vi "CRake Learn Template.vi"(8 "error in":errorcluster, 9 "Image in":T1, 10 "Template details":T2={"Process parameters"={"ROI parameters"={"Step Size"=20, "r offset"=10, "Edge Options"={"Edge Polarity"=0, "Kernel Size"=7, "Width"=5, "Minimum Edge Strength"=100.0, "Interpolation Type"=enum."Bilinear Fixed", "Data Processing Method"=enum."Average"}, "Annulus\ndetails"={"Center X"=0, "Center Y"=0, "Inner Radius"=0, "Outer Radius"=3900, "Start Angle"=0.0, "End Angle"=0.0}}, "Dust removal details"={"Remove dust"=TRUE, "Dust removal data"={"Dilate data"={"Operation"=enum."Erode", "Structuring Element"=[[1, 1, 1], [1, 1, 1], [1, 1, 1]], "Number of iterations (1)"=3, "Square/Hexa (Square)"=TRUE}, "Threshold data"={"Method (clustering)"=0, "Look For (Bright Objects)"=1, "Range"={"Lower value"=128.0, "Upper value"=255.0}, "Replace Value"=255.0}}}}, "LearningData"={"Angle info"={"Rising edge angles"=[{"Edge angles"=[]}, {"Edge angles"=[]}, {"Edge angles"=[]}, {"Edge angles"=[]}, {"Edge angles"=[]}, {"Edge angles"=[]}, {"Edge angles"=[]}, {"Edge angles"=[]}, {"Edge angles"=[]}, {"Edge angles"=[]}, {"Edge angles"=[]}, {"Edge angles"=[]}, {"Edge angles"=[]}, {"Edge angles"=[]}, {"Edge angles"=[324.4002990722656, 279.37237548828125, 234.31814575195312, 189.45828247070312, 144.43719482421875, 99.26164245605469, 54.478885650634766, 9.288665771484375]}, {"Edge angles"=[326.8953857421875, 282.0519714355469, 237.04156494140625, 192.0699920654297, 147.00604248046875, 102.04810333251953, 57.04718017578125, 12.020856857299805]}, {"Edge angles"=[327.23541259765625, 282.35137939453125, 237.37074279785156, 192.36749267578125, 147.3665313720703, 102.35699462890625, 57.358543395996094, 12.353824615478516]}, {"Edge angles"=[357.3017883300781, 326.07904052734375, 281.0994567871094, 236.0724639892578, 235.6566925048828, 191.1215057373047, 146.08834838867188, 101.15013122558594, 56.03056716918945, 11.077372550964355]}, {"Edge angles"=[322.224609375, 277.2630615234375, 232.26690673828125, 96.92642974853516, 52.116703033447266, 7.029767990112305]}, {"Edge angles"=[]}, {"Edge angles"=[]}, {"Edge angles"=[]}, {"Edge angles"=[]}, {"Edge angles"=[]}, {"Edge angles"=[]}, {"Edge angles"=[]}, {"Edge angles"=[356.58099365234375, 350.285400390625, 343.9516296386719, 337.64874267578125, 331.33636474609375, 325.0185241699219, 318.6827697753906, 312.3748779296875, 306.0724792480469, 299.736083984375, 293.4723815917969, 287.15020751953125, 280.8420715332031, 274.51861572265625, 268.1320495605469, 261.8740539550781, 255.5738983154297, 249.276123046875, 242.95098876953125, 236.62612915039062, 230.31637573242188, 224.009521484375, 217.69149780273438, 211.35440063476562, 205.0513916015625, 198.69039916992188, 192.43421936035156, 186.09483337402344, 179.81744384765625, 173.4593505859375, 167.0970001220703, 160.7847900390625, 154.46017456054688, 148.13107299804688, 141.8062286376953, 135.53399658203125, 129.20545959472656, 122.88826751708984, 116.5517349243164, 110.27731323242188, 103.95439910888672, 97.63215637207031, 91.3005142211914, 85.0173568725586, 78.71366119384766, 72.41765594482422, 65.96402740478516, 59.750633239746094, 53.4320068359375, 47.08340835571289, 40.791725158691406, 34.49047088623047, 28.16463851928711, 21.869430541992188, 15.541481018066406, 9.238995552062988, 2.9198527336120605]}, {"Edge angles"=[357.50360107421875, 351.15313720703125, 344.8380432128906, 338.5302429199219, 332.2137756347656, 325.804443359375, 319.57830810546875, 313.2322998046875, 306.92938232421875, 300.63079833984375, 294.3407287597656, 288.0224304199219, 281.7042236328125, 275.3729248046875, 269.0707702636719, 262.775390625, 256.4610900878906, 250.14210510253906, 243.842529296875, 237.52635192871094, 231.20989990234375, 224.88641357421875, 218.57626342773438, 212.2597198486328, 205.92007446289062, 199.60572814941406, 193.28834533691406, 186.9896240234375, 180.66493225097656, 174.3603057861328, 168.0143280029297, 161.70201110839844, 155.35635375976562, 149.0479278564453, 142.74942016601562, 136.41973876953125, 130.07635498046875, 123.77355194091797, 117.44210815429688, 111.15596771240234, 104.81024932861328, 98.50434875488281, 92.1738510131836, 85.8763427734375, 79.58023071289062, 73.2815170288086, 66.96917724609375, 60.62763595581055, 54.32320785522461, 48.03331756591797, 41.69807434082031, 35.39656066894531, 29.04926872253418, 22.751008987426758, 16.438982009887695, 10.120953559875488, 3.7855653762817383]}], "Falling edge angles"=[{"Edge angles"=[]}, {"Edge angles"=[]}, {"Edge angles"=[]}, {"Edge angles"=[]}, {"Edge angles"=[]}, {"Edge angles"=[]}, {"Edge angles"=[]}, {"Edge angles"=[]}, {"Edge angles"=[]}, {"Edge angles"=[]}, {"Edge angles"=[]}, {"Edge angles"=[]}, {"Edge angles"=[]}, {"Edge angles"=[]}, {"Edge angles"=[358.7027587890625, 313.5650939941406, 268.6748962402344, 223.70919799804688, 178.54701232910156, 133.67933654785156, 88.60447692871094, 43.56612777709961]}, {"Edge angles"=[355.9402770996094, 310.9671325683594, 266.03912353515625, 221.030029296875, 175.98460388183594, 130.972412109375, 86.0030517578125, 40.94852828979492]}, {"Edge angles"=[355.5914611816406, 310.6212463378906, 265.676513671875, 220.6667022705078, 175.67599487304688, 130.68984985351562, 85.72019958496094, 40.68776321411133]}, {"Edge angles"=[357.8193054199219, 357.139404296875, 311.851318359375, 266.9569091796875, 235.827880859375, 221.9400177001953, 176.938232421875, 131.88555908203125, 86.9477310180664, 41.9368782043457]}, {"Edge angles"=[315.7031555175781, 225.93267822265625, 180.75328063964844, 135.82232666015625, 46.085636138916016, 0.9171632528305054]}, {"Edge angles"=[]}, {"Edge angles"=[]}, {"Edge angles"=[]}, {"Edge angles"=[]}, {"Edge angles"=[]}, {"Edge angles"=[]}, {"Edge angles"=[]}, {"Edge angles"=[354.0222473144531, 347.68878173828125, 341.4031677246094, 335.0976257324219, 328.770263671875, 322.4639892578125, 316.15887451171875, 309.8772277832031, 303.5346984863281, 297.2074890136719, 290.9279479980469, 284.62744140625, 278.2616882324219, 271.9461669921875, 265.6507568359375, 259.335205078125, 253.01336669921875, 246.688720703125, 240.3791961669922, 234.10598754882812, 227.7845001220703, 221.4361114501953, 215.10934448242188, 208.79022216796875, 202.47589111328125, 196.1585235595703, 189.9136505126953, 183.51986694335938, 177.2025604248047, 170.8728485107422, 164.5511932373047, 158.22274780273438, 151.91403198242188, 145.59686279296875, 139.29791259765625, 132.97251892089844, 126.62997436523438, 120.33435821533203, 114.02253723144531, 107.7345199584961, 101.3875503540039, 95.11666107177734, 88.78436279296875, 82.45806884765625, 76.13545227050781, 69.85616302490234, 63.47029113769531, 57.14175796508789, 50.845458984375, 44.541873931884766, 38.223140716552734, 31.949254989624023, 25.62628746032715, 19.294870376586914, 12.989399909973145, 6.6459808349609375, 0.32935503125190735]}, {"Edge angles"=[359.45294189453125, 353.155517578125, 346.8225402832031, 340.52154541015625, 334.2013854980469, 327.8995361328125, 321.5911865234375, 315.29925537109375, 308.96868896484375, 302.6675720214844, 296.33758544921875, 290.021728515625, 283.70550537109375, 277.3900451660156, 271.0820007324219, 264.7945556640625, 258.4638366699219, 252.13612365722656, 245.82635498046875, 239.5060272216797, 233.20834350585938, 226.8910675048828, 220.53424072265625, 214.2158203125, 207.89846801757812, 201.5936279296875, 195.26161193847656, 188.94100952148438, 182.6217803955078, 176.31558227539062, 169.99583435058594, 163.67674255371094, 157.3478240966797, 151.02032470703125, 144.70858764648438, 138.41078186035156, 132.12911987304688, 125.7828140258789, 119.45489501953125, 113.16563415527344, 106.87589263916016, 100.5637435913086, 94.23698425292969, 87.91885375976562, 81.59281921386719, 75.27478790283203, 68.95628356933594, 62.62395477294922, 56.29034423828125, 49.94796371459961, 43.6364631652832, 37.34098815917969, 31.032493591308594, 24.706125259399414, 18.384830474853516, 12.063972473144531, 5.750241279602051]}]}, "Center"={"X"=5341.767, "Y"=4601.92}}, "Fine search details"={"FS angle range\n(in degrees)"=5.0, "FS angle step size\n(in degrees)"=0.001}, "Auto ROI detect"=TRUE} {"Process parameters"."ROI parameters"."Edge Options"."Edge Polarity" items=["All Edges", "Rising Edges", "Falling Edges"]; "Process parameters"."ROI parameters"."Edge Options"."Minimum Edge Strength" format="%.2f"; "Process parameters"."ROI parameters"."Edge Options"."Width" step=2; "Process parameters"."ROI parameters"."Edge Options"."Kernel Size" step=2; "Process parameters"."ROI parameters"."Annulus\ndetails"."End Angle" min=-90.0 max=90.0 step=1.0 format="%.2f"; "Process parameters"."ROI parameters"."Annulus\ndetails"."Start Angle" min=-90.0 max=90.0 step=1.0 format="%.2f"; "Process parameters"."ROI parameters"."Annulus\ndetails"."Center X" scale=0.0..1024.0; "Process parameters"."Dust removal details"."Dust removal data"."Threshold data"."Method (clustering)" items=["clustering", "entropy", "metric", "moments", "inter-class variance"]; "Process parameters"."Dust removal details"."Dust removal data"."Threshold data"."Look For (Bright Objects)" items=["Bright Objects", "Dark Objects"]}, 11 "Write parameters":T7={"Part name"="", "TemplateImage filepath"=path "E:/Algorithm/Geometric template matching/Images/Test images/Partially symmetric part/Part 1/Coarse angle/41.000000.png", "Template config filepath"=path "", "Testing?"=FALSE}) -> (0 "error out":errorcluster, 2 "Image indicator":T1(plugin-control), 3 "Template details out":T2={"Process parameters"={"ROI parameters"={"Step Size"=75, "r offset"=0, "Edge Options"={"Edge Polarity"=0, "Kernel Size"=0, "Width"=10, "Minimum Edge Strength"=2800.0, "Interpolation Type"=enum."Zero Order", "Data Processing Method"=enum."Average"}, "Annulus\ndetails"={"Center X"=0, "Center Y"=0, "Inner Radius"=0, "Outer Radius"=0, "Start Angle"=0.0, "End Angle"=0.0}}, "Dust removal details"={"Remove dust"=FALSE, "Dust removal data"={"Dilate data"={"Operation"=enum."Erode", "Structuring Element"=[[1, 1, 1], [1, 1, 1], [1, 1, 1]], "Number of iterations (1)"=5, "Square/Hexa (Square)"=TRUE}, "Threshold data"={"Method (clustering)"=0, "Look For (Bright Objects)"=1, "Range"={"Lower value"=128.0, "Upper value"=255.0}, "Replace Value"=255.0}}}}, "LearningData"={"Angle info"={"Rising edge angles"=[{"Edge angles"=[]}, {"Edge angles"=[]}, {"Edge angles"=[]}, {"Edge angles"=[]}, {"Edge angles"=[]}, {"Edge angles"=[]}, {"Edge angles"=[]}, {"Edge angles"=[]}, {"Edge angles"=[]}, {"Edge angles"=[]}, {"Edge angles"=[]}, {"Edge angles"=[]}, {"Edge angles"=[]}, {"Edge angles"=[]}, {"Edge angles"=[324.4002990722656, 279.37237548828125, 234.31814575195312, 189.45828247070312, 144.43719482421875, 99.26164245605469, 54.478885650634766, 9.288665771484375]}, {"Edge angles"=[326.8953857421875, 282.0519714355469, 237.04156494140625, 192.0699920654297, 147.00604248046875, 102.04810333251953, 57.04718017578125, 12.020856857299805]}, {"Edge angles"=[327.23541259765625, 282.35137939453125, 237.37074279785156, 192.36749267578125, 147.3665313720703, 102.35699462890625, 57.358543395996094, 12.353824615478516]}, {"Edge angles"=[357.3017883300781, 326.07904052734375, 281.0994567871094, 236.0724639892578, 235.6566925048828, 191.1215057373047, 146.08834838867188, 101.15013122558594, 56.03056716918945, 11.077372550964355]}, {"Edge angles"=[322.224609375, 277.2630615234375, 232.26690673828125, 96.92642974853516, 52.116703033447266, 7.029767990112305]}, {"Edge angles"=[]}, {"Edge angles"=[]}, {"Edge angles"=[]}, {"Edge angles"=[]}, {"Edge angles"=[]}, {"Edge angles"=[]}, {"Edge angles"=[]}, {"Edge angles"=[356.58099365234375, 350.285400390625, 343.9516296386719, 337.64874267578125, 331.33636474609375, 325.0185241699219, 318.6827697753906, 312.3748779296875, 306.0724792480469, 299.736083984375, 293.4723815917969, 287.15020751953125, 280.8420715332031, 274.51861572265625, 268.1320495605469, 261.8740539550781, 255.5738983154297, 249.276123046875, 242.95098876953125, 236.62612915039062, 230.31637573242188, 224.009521484375, 217.69149780273438, 211.35440063476562, 205.0513916015625, 198.69039916992188, 192.43421936035156, 186.09483337402344, 179.81744384765625, 173.4593505859375, 167.0970001220703, 160.7847900390625, 154.46017456054688, 148.13107299804688, 141.8062286376953, 135.53399658203125, 129.20545959472656, 122.88826751708984, 116.5517349243164, 110.27731323242188, 103.95439910888672, 97.63215637207031, 91.3005142211914, 85.0173568725586, 78.71366119384766, 72.41765594482422, 65.96402740478516, 59.750633239746094, 53.4320068359375, 47.08340835571289, 40.791725158691406, 34.49047088623047, 28.16463851928711, 21.869430541992188, 15.541481018066406, 9.238995552062988, 2.9198527336120605]}, {"Edge angles"=[357.50360107421875, 351.15313720703125, 344.8380432128906, 338.5302429199219, 332.2137756347656, 325.804443359375, 319.57830810546875, 313.2322998046875, 306.92938232421875, 300.63079833984375, 294.3407287597656, 288.0224304199219, 281.7042236328125, 275.3729248046875, 269.0707702636719, 262.775390625, 256.4610900878906, 250.14210510253906, 243.842529296875, 237.52635192871094, 231.20989990234375, 224.88641357421875, 218.57626342773438, 212.2597198486328, 205.92007446289062, 199.60572814941406, 193.28834533691406, 186.9896240234375, 180.66493225097656, 174.3603057861328, 168.0143280029297, 161.70201110839844, 155.35635375976562, 149.0479278564453, 142.74942016601562, 136.41973876953125, 130.07635498046875, 123.77355194091797, 117.44210815429688, 111.15596771240234, 104.81024932861328, 98.50434875488281, 92.1738510131836, 85.8763427734375, 79.58023071289062, 73.2815170288086, 66.96917724609375, 60.62763595581055, 54.32320785522461, 48.03331756591797, 41.69807434082031, 35.39656066894531, 29.04926872253418, 22.751008987426758, 16.438982009887695, 10.120953559875488, 3.7855653762817383]}], "Falling edge angles"=[{"Edge angles"=[]}, {"Edge angles"=[]}, {"Edge angles"=[]}, {"Edge angles"=[]}, {"Edge angles"=[]}, {"Edge angles"=[]}, {"Edge angles"=[]}, {"Edge angles"=[]}, {"Edge angles"=[]}, {"Edge angles"=[]}, {"Edge angles"=[]}, {"Edge angles"=[]}, {"Edge angles"=[]}, {"Edge angles"=[]}, {"Edge angles"=[358.7027587890625, 313.5650939941406, 268.6748962402344, 223.70919799804688, 178.54701232910156, 133.67933654785156, 88.60447692871094, 43.56612777709961]}, {"Edge angles"=[355.9402770996094, 310.9671325683594, 266.03912353515625, 221.030029296875, 175.98460388183594, 130.972412109375, 86.0030517578125, 40.94852828979492]}, {"Edge angles"=[355.5914611816406, 310.6212463378906, 265.676513671875, 220.6667022705078, 175.67599487304688, 130.68984985351562, 85.72019958496094, 40.68776321411133]}, {"Edge angles"=[357.8193054199219, 357.139404296875, 311.851318359375, 266.9569091796875, 235.827880859375, 221.9400177001953, 176.938232421875, 131.88555908203125, 86.9477310180664, 41.9368782043457]}, {"Edge angles"=[315.7031555175781, 225.93267822265625, 180.75328063964844, 135.82232666015625, 46.085636138916016, 0.9171632528305054]}, {"Edge angles"=[]}, {"Edge angles"=[]}, {"Edge angles"=[]}, {"Edge angles"=[]}, {"Edge angles"=[]}, {"Edge angles"=[]}, {"Edge angles"=[]}, {"Edge angles"=[354.0222473144531, 347.68878173828125, 341.4031677246094, 335.0976257324219, 328.770263671875, 322.4639892578125, 316.15887451171875, 309.8772277832031, 303.5346984863281, 297.2074890136719, 290.9279479980469, 284.62744140625, 278.2616882324219, 271.9461669921875, 265.6507568359375, 259.335205078125, 253.01336669921875, 246.688720703125, 240.3791961669922, 234.10598754882812, 227.7845001220703, 221.4361114501953, 215.10934448242188, 208.79022216796875, 202.47589111328125, 196.1585235595703, 189.9136505126953, 183.51986694335938, 177.2025604248047, 170.8728485107422, 164.5511932373047, 158.22274780273438, 151.91403198242188, 145.59686279296875, 139.29791259765625, 132.97251892089844, 126.62997436523438, 120.33435821533203, 114.02253723144531, 107.7345199584961, 101.3875503540039, 95.11666107177734, 88.78436279296875, 82.45806884765625, 76.13545227050781, 69.85616302490234, 63.47029113769531, 57.14175796508789, 50.845458984375, 44.541873931884766, 38.223140716552734, 31.949254989624023, 25.62628746032715, 19.294870376586914, 12.989399909973145, 6.6459808349609375, 0.32935503125190735]}, {"Edge angles"=[359.45294189453125, 353.155517578125, 346.8225402832031, 340.52154541015625, 334.2013854980469, 327.8995361328125, 321.5911865234375, 315.29925537109375, 308.96868896484375, 302.6675720214844, 296.33758544921875, 290.021728515625, 283.70550537109375, 277.3900451660156, 271.0820007324219, 264.7945556640625, 258.4638366699219, 252.13612365722656, 245.82635498046875, 239.5060272216797, 233.20834350585938, 226.8910675048828, 220.53424072265625, 214.2158203125, 207.89846801757812, 201.5936279296875, 195.26161193847656, 188.94100952148438, 182.6217803955078, 176.31558227539062, 169.99583435058594, 163.67674255371094, 157.3478240966797, 151.02032470703125, 144.70858764648438, 138.41078186035156, 132.12911987304688, 125.7828140258789, 119.45489501953125, 113.16563415527344, 106.87589263916016, 100.5637435913086, 94.23698425292969, 87.91885375976562, 81.59281921386719, 75.27478790283203, 68.95628356933594, 62.62395477294922, 56.29034423828125, 49.94796371459961, 43.6364631652832, 37.34098815917969, 31.032493591308594, 24.706125259399414, 18.384830474853516, 12.063972473144531, 5.750241279602051]}]}, "Center"={"X"=5341.767, "Y"=4601.92}}, "Fine search details"={"FS angle range\n(in degrees)"=5.0, "FS angle step size\n(in degrees)"=0.01}, "Auto ROI detect"=TRUE} {"Process parameters"."ROI parameters"."Edge Options"."Edge Polarity" items=["All Edges", "Rising Edges", "Falling Edges"]; "Process parameters"."ROI parameters"."Edge Options"."Minimum Edge Strength" format="%.2f"; "Process parameters"."ROI parameters"."Edge Options"."Width" step=2; "Process parameters"."ROI parameters"."Edge Options"."Kernel Size" step=2; "Process parameters"."ROI parameters"."Annulus\ndetails"."End Angle" min=-90.0 max=90.0 step=1.0 format="%.2f"; "Process parameters"."ROI parameters"."Annulus\ndetails"."Start Angle" min=-90.0 max=90.0 step=1.0 format="%.2f"; "Process parameters"."ROI parameters"."Annulus\ndetails"."Center X" scale=0.0..1024.0; "Process parameters"."Dust removal details"."Dust removal data"."Threshold data"."Method (clustering)" items=["clustering", "entropy", "metric", "moments", "inter-class variance"]; "Process parameters"."Dust removal details"."Dust removal data"."Threshold data"."Look For (Bright Objects)" items=["Bright Objects", "Dark Objects"]})   [LabVIEW 2015]
uses:
  CRake Pattern Matching/Controls/JSON parameters.ctl
  CRake Pattern Matching/Controls/ROI parameters.ctl
  <vilib>/vision/Measure.llb/Edge Options.ctl
  <vilib>/vision/Measure.llb/Edge Polarity.ctl
  <vilib>/vision/Image Controls.llb/IMAQ Image.ctl
panel:
  out "Image indicator 2":T1(plugin-control)
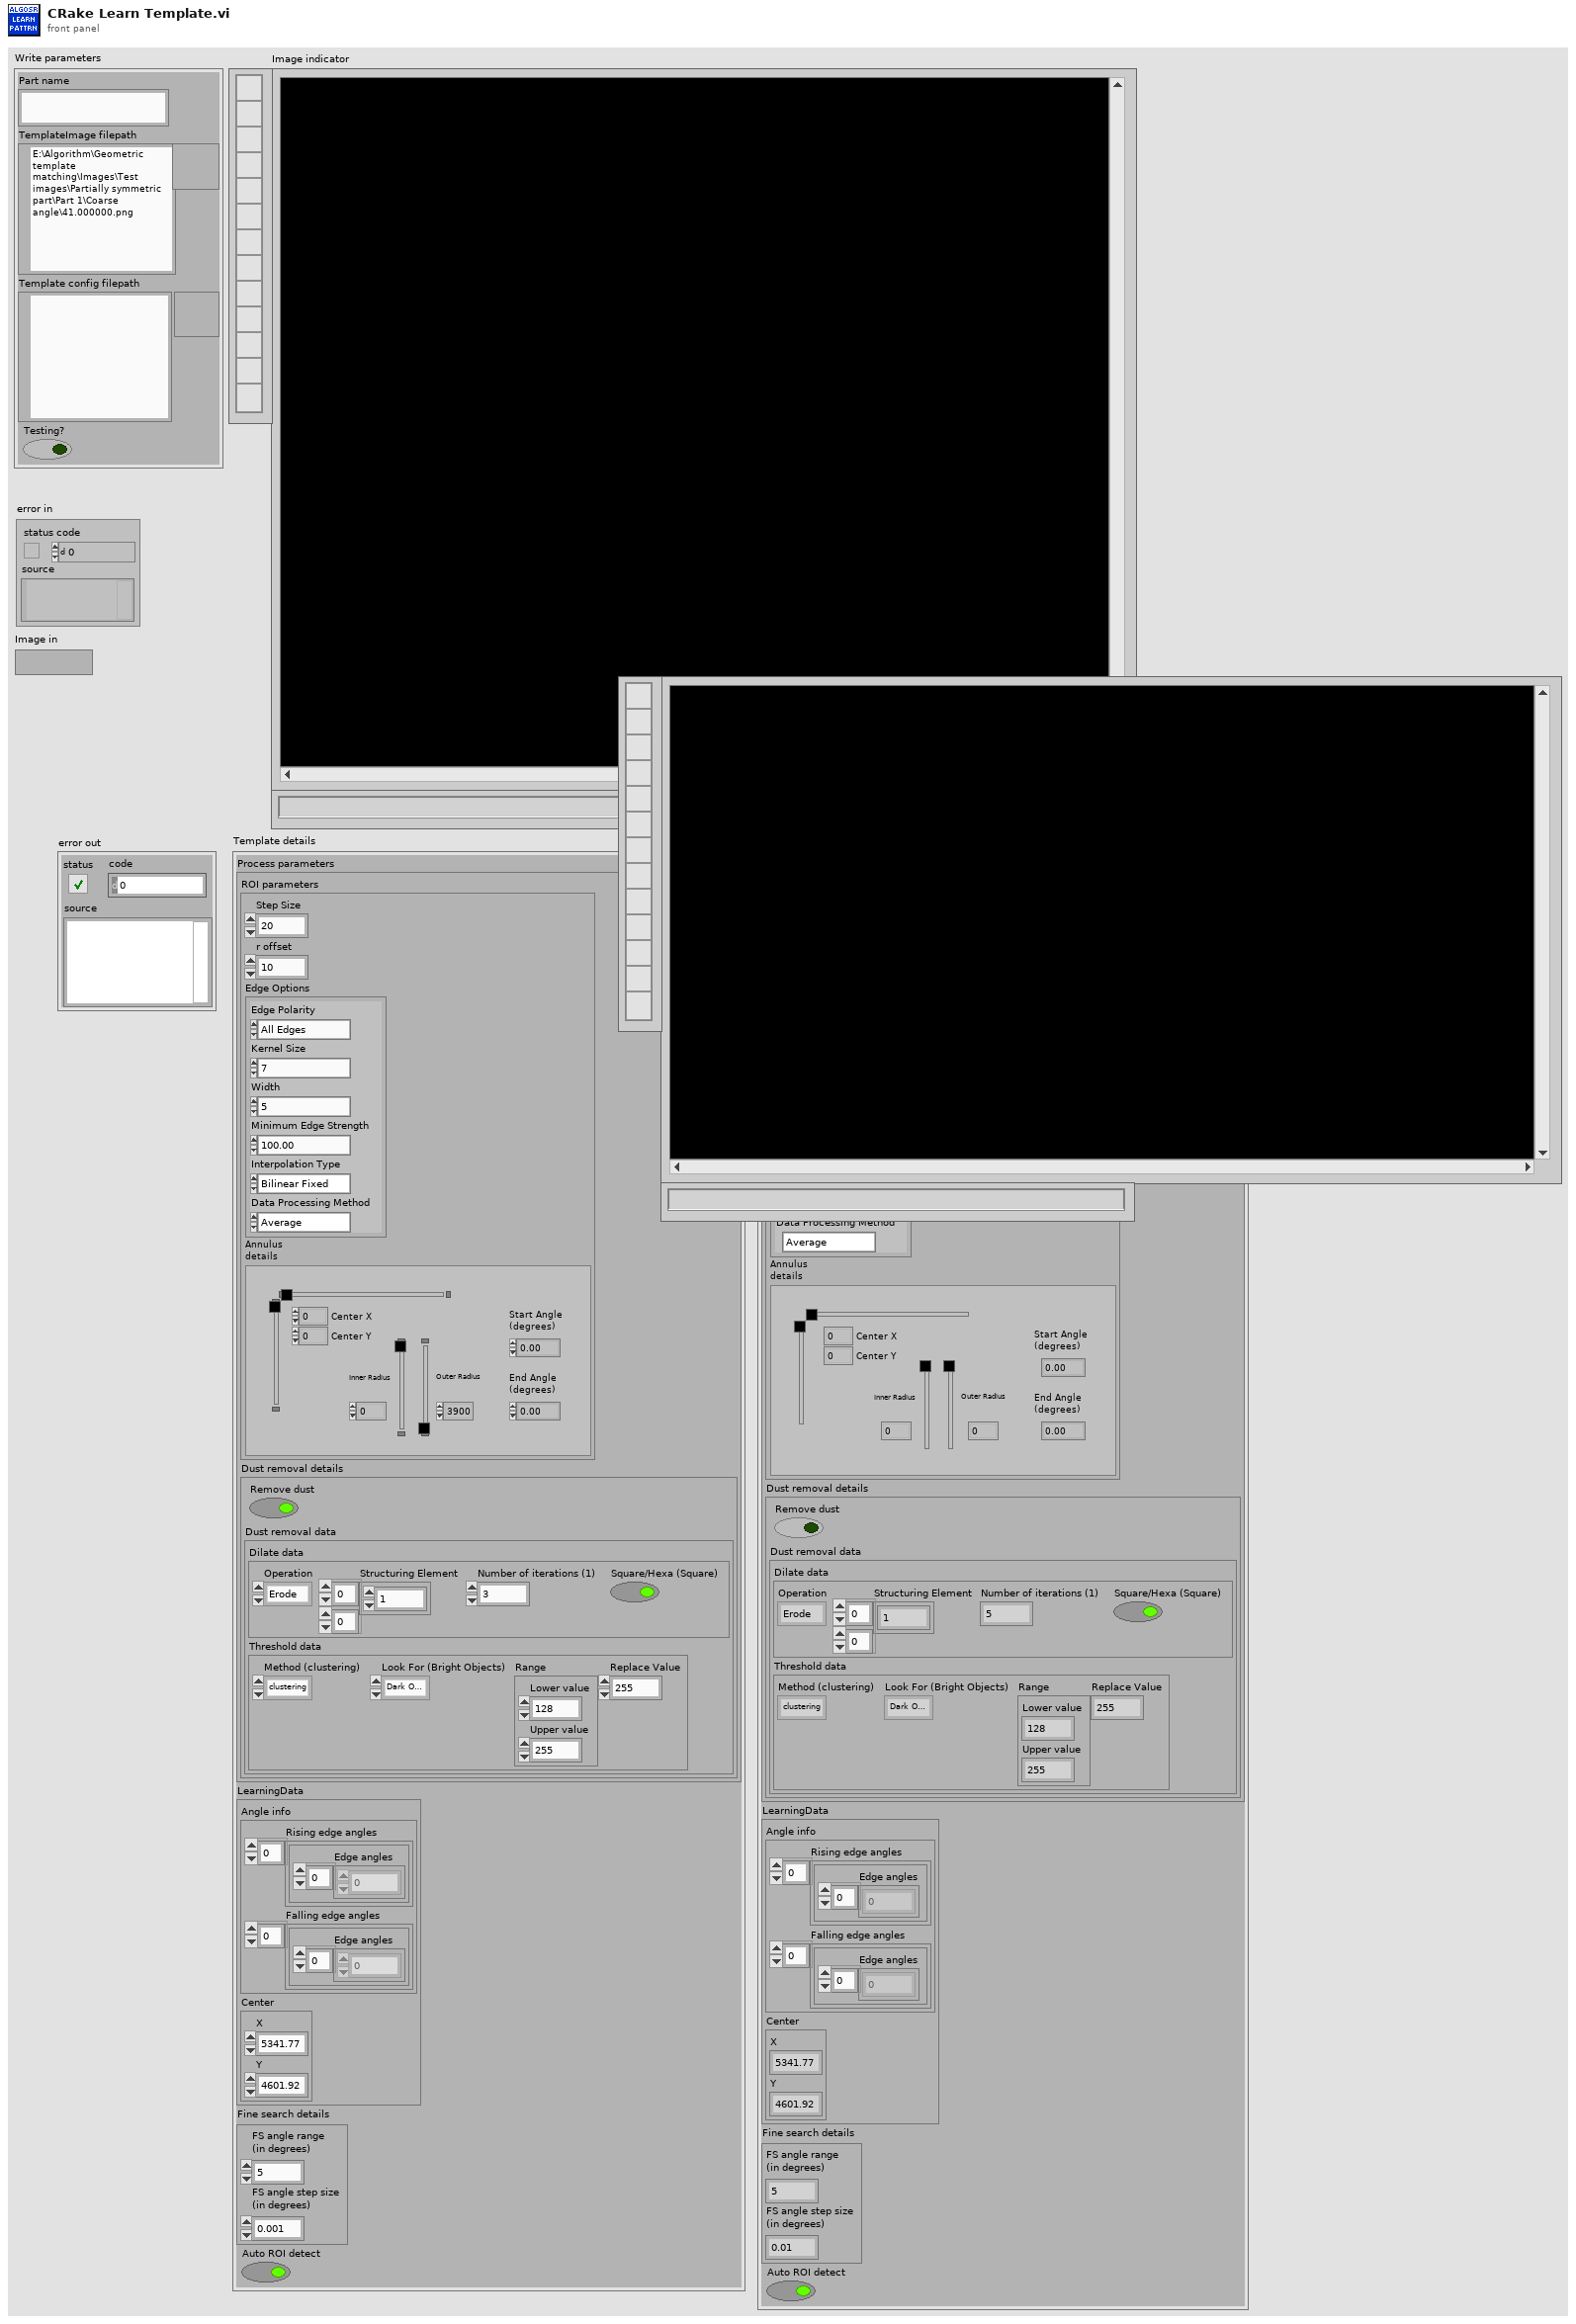
[diagram p1: front panel]
types:
  T1 = typedef "IMAQ Image.ctl" = refnum<image>
  T2 = typedef "JSON parameters.ctl" = cluster{"Process parameters":cluster{"ROI parameters":T3, "Dust removal details":cluster{"Remove dust":bool, "Dust removal data":cluster{"Dilate data":cluster{"Operation":enum32{"AutoM", "Close", "Dilate", "Erode", "Gradient", "Gradient out", "Gradient in", "Hit miss", "Open", "PClose", "POpen", "Thick", "Thin"}, "Structuring Element":i32[][], "Number of iterations (1)":i32, "Square/Hexa (Square)":bool}, "Threshold data":cluster{"Method (clustering)":i32, "Look For (Bright Objects)":u32, "Range":cluster{"Lower value":sgl, "Upper value":sgl}, "Replace Value":sgl}}}}, "LearningData":cluster{"Angle info":cluster{"Rising edge angles":cluster{"Edge angles":dbl[]}[], "Falling edge angles":cluster{"Edge angles":dbl[]}[]}, "Center":cluster{"X":sgl, "Y":sgl}}, "Fine search details":cluster{"FS angle range\n(in degrees)":dbl, "FS angle step size\n(in degrees)":dbl}, "Auto ROI detect":bool}
  T3 = typedef "ROI parameters.ctl" = cluster{"Step Size":u32, "r offset":u32, "Edge Options":T4, "Annulus\ndetails":T6}
  T4 = typedef "Edge Options.ctl" = cluster{"Edge Polarity":T5, "Kernel Size":u32, "Width":u32, "Minimum Edge Strength":sgl, "Interpolation Type":enum32{"Zero Order", "Bilinear", "Quadratic", "Cubic", "Bilinear Fixed"}, "Data Processing Method":enum32{"Average", "Median"}}
  T5 = typedef "Edge Polarity.ctl" = u32
  T6 = typedef "IMAQ Circle" = cluster{"Center X":i32, "Center Y":i32, "Inner Radius":i32, "Outer Radius":i32, "Start Angle":dbl, "End Angle":dbl}
  T7 = cluster{"Part name":string, "TemplateImage filepath":path, "Template config filepath":path, "Testing?":bool}
  T8 = cluster{"FS angle range\n(in degrees)":dbl, "FS angle step size\n(in degrees)":dbl}
  T9 = cluster{"Remove dust":bool, "Dust removal data":cluster{"Dilate data":cluster{"Operation":enum32{"AutoM", "Close", "Dilate", "Erode", "Gradient", "Gradient out", "Gradient in", "Hit miss", "Open", "PClose", "POpen", "Thick", "Thin"}, "Structuring Element":i32[][], "Number of iterations (1)":i32, "Square/Hexa (Square)":bool}, "Threshold data":cluster{"Method (clustering)":i32, "Look For (Bright Objects)":u32, "Range":cluster{"Lower value":sgl, "Upper value":sgl}, "Replace Value":sgl}}}
  T10 = cluster{"Dilate data":cluster{"Operation":enum32{"AutoM", "Close", "Dilate", "Erode", "Gradient", "Gradient out", "Gradient in", "Hit miss", "Open", "PClose", "POpen", "Thick", "Thin"}, "Structuring Element":i32[][], "Number of iterations (1)":i32, "Square/Hexa (Square)":bool}, "Threshold data":cluster{"Method (clustering)":i32, "Look For (Bright Objects)":u32, "Range":cluster{"Lower value":sgl, "Upper value":sgl}, "Replace Value":sgl}}
  T11 = cluster{"Angle info":cluster{"Rising edge angles":cluster{"Edge angles":dbl[]}[], "Falling edge angles":cluster{"Edge angles":dbl[]}[]}, "Center":cluster{"X":sgl, "Y":sgl}}
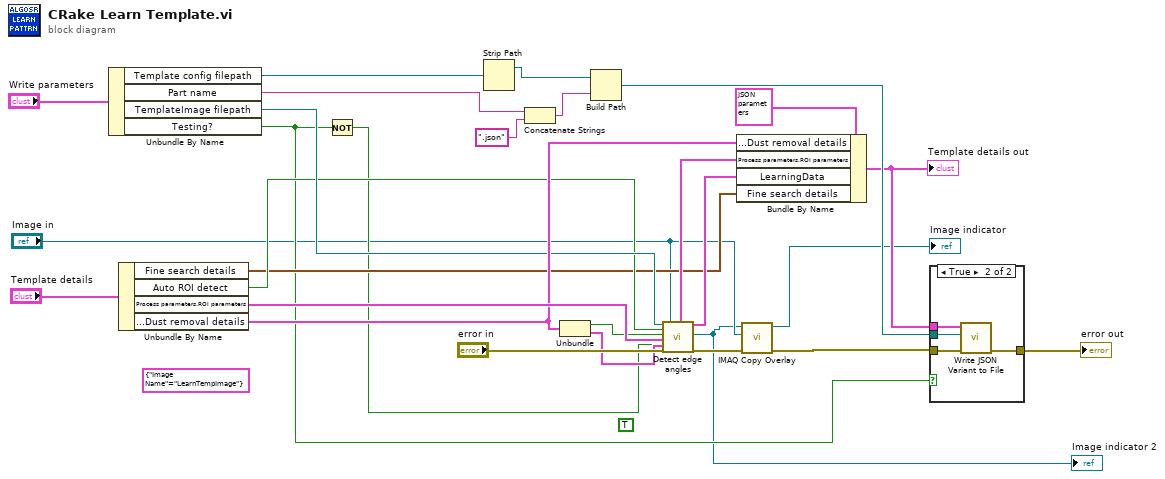
[diagram p0: block diagram]
diagram:
  (unwired) cluster{"Image Name":string} {"Image Name"="LearnTempImage"} ("BufferData")
  (unwired) TRUE ("Overlay?")
  n1 = Unbundle By Name("Write parameters") -> ("Template config filepath"=w11:path, "Part name"=w12:string, "TemplateImage filepath"=w10:path, "Testing?"=w7:bool)
  n2 = Unbundle By Name("Template details") -> ("Fine search details"=w8:T8, "Auto ROI detect"=w9:bool, "Process parameters.ROI parameters"=w22:T3, "Process parameters.Dust removal details"=w16:T9)
  n3 = Not(x=w7) -> (.not. x?=w6:bool)
  n4 = Strip Path(path=w11) -> (stripped path=w23:path)  [unwired: 1 out]
  n5 = Concatenate Strings(w12, ".json" ("string")) -> (w25:string)
  n6 = Unbundle(w16) -> ("Remove dust"=w21:bool, "Dust removal data"=w20:T10)
  n7 = Build Path(base path=w23, name or relative path=w25) -> (appended path=w24:path)
  n8 = call "Detect edge angles.vi"("Image filepath"=w10, "Auto ROI detect"=w9, "Remove dust?"=w21, "ROI parameters\nFeature"=w22, "Image input?"=w6, "error in"="error in", "Image in"="Image in", "Dust removal data"=w20) -> ("ROI parameters\nFeature out"=w17:T3, "Output"=w18:T11, "Image indicator"=w1:T1, "error out"=w5:errorcluster)  [unwired: 8 in]
  "Image indicator 2" <- w1
  n9 = Bundle By Name(cluster=T2 {"Process parameters"={"ROI parameters"={"Step Size"=80, "r offset"=0, "Edge Options"={"Edge Polarity"=0, "Kernel Size"=0, "Width"=10, "Minimum Edge Strength"=3700.0, "Interpolation Type"=enum."Zero Order", "Data Processing Method"=enum."Average"}, "Annulus\ndetails"={"Center X"=0, "Center Y"=0, "Inner Radius"=0, "Outer Radius"=0, "Start Angle"=0.0, "End Angle"=0.0}}, "Dust removal details"={"Remove dust"=TRUE, "Dust removal data"={"Dilate data"={"Operation"=enum."Erode", "Structuring Element"=[[1, 1, 1], [1, 1, 1], [1, 1, 1]], "Number of iterations (1)"=5, "Square/Hexa (Square)"=TRUE}, "Threshold data"={"Method (clustering)"=0, "Look For (Bright Objects)"=1, "Range"={"Lower value"=128.0, "Upper value"=255.0}, "Replace Value"=1.0}}}}, "LearningData"={"Angle info"={"Rising edge angles"=[{"Edge angles"=[]}, {"Edge angles"=[]}, {"Edge angles"=[]}, {"Edge angles"=[354.382568359375, 295.7427062988281, 72.67430877685547]}, {"Edge angles"=[]}, {"Edge angles"=[]}, {"Edge angles"=[315.599609375, 135.69708251953125]}, {"Edge angles"=[314.0948181152344, 134.1259307861328]}, {"Edge angles"=[]}, {"Edge angles"=[]}, {"Edge angles"=[]}, {"Edge angles"=[342.3753662109375, 316.6233215332031, 290.9537658691406, 265.174072265625, 239.4954833984375, 212.9640655517578, 187.85411071777344, 162.35777282714844, 136.55381774902344, 110.95350646972656, 85.18316650390625, 59.44724655151367, 33.712345123291016, 7.991258144378662]}, {"Edge angles"=[345.2440490722656, 319.5457458496094, 293.83245849609375, 268.09527587890625, 242.34674072265625, 216.6270294189453, 190.92391967773438, 165.19166564941406, 139.54507446289062, 113.81599426269531, 88.05338287353516, 62.330039978027344, 36.62122344970703, 10.95604419708252]}, {"Edge angles"=[346.6121826171875, 320.9537048339844, 295.2318115234375, 269.4681701660156, 243.7433319091797, 218.04986572265625, 192.27938842773438, 166.63919067382812, 140.93756103515625, 115.16751861572266, 89.4376220703125, 63.72598648071289, 37.99089431762695, 12.334281921386719]}, {"Edge angles"=[]}], "Falling edge angles"=[{"Edge angles"=[]}, {"Edge angles"=[]}, {"Edge angles"=[]}, {"Edge angles"=[355.8258361816406, 316.2864990234375, 256.6278381347656, 76.5568618774414, 74.29270935058594, 68.8586654663086, 16.1683406829834]}, {"Edge angles"=[]}, {"Edge angles"=[]}, {"Edge angles"=[296.0315246582031, 115.80548858642578]}, {"Edge angles"=[297.45526123046875, 117.18331909179688]}, {"Edge angles"=[]}, {"Edge angles"=[]}, {"Edge angles"=[]}, {"Edge angles"=[354.8468017578125, 329.16796875, 303.61322021484375, 277.72528076171875, 251.94198608398438, 226.30845642089844, 200.55133056640625, 174.85848999023438, 149.2189483642578, 123.45135498046875, 97.71527862548828, 71.9430160522461, 46.20140838623047, 20.491928100585938]}, {"Edge angles"=[351.9039611816406, 326.2618103027344, 300.5503234863281, 274.89703369140625, 249.1070556640625, 223.36106872558594, 197.6668243408203, 171.93382263183594, 146.27853393554688, 120.5433120727539, 94.8203125, 69.03418731689453, 43.36899948120117, 17.62021827697754]}, {"Edge angles"=[350.552490234375, 324.9085693359375, 299.203857421875, 273.4911804199219, 247.75616455078125, 221.9854736328125, 196.28067016601562, 170.53329467773438, 144.81431579589844, 119.17356872558594, 93.42098999023438, 67.66309356689453, 41.889286041259766, 16.27904510498047]}, {"Edge angles"=[]}]}, "Center"={"X"=1145.5413, "Y"=1999.3091}}, "Fine search details"={"FS angle range\n(in degrees)"=5.0, "FS angle step size\n(in degrees)"=0.01}, "Auto ROI detect"=TRUE} ("JSON parameters"), "Process parameters.Dust removal details"=w16, "Process parameters.ROI parameters"=w17, "LearningData"=w18, "Fine search details"=w8) -> (w14:T2)
  "Template details out" <- w14
  n10 = call "IMAQ Copy Overlay"("error in (no error)"=w5, "Image Dst"="Image in", "Image Src"=w1) -> ("error out"=w2:errorcluster, "Image Dst Out"=→"Image indicator":T1)  [unwired: 7 in]
  n11 = case shown="True" w7 {
    tunnel: [w29 w33] -> w27
    tunnel: w24 -> [_ w32]
    tunnel: w2 -> [w29 w31]
    tunnel: w14 -> [_ w30]
    frame False {
    }
    frame True {
      n12 = call <vilib>:"Write JSON Variant to File.vi"("Error In"=w31, "file (use dialog)"=w32, "JSON Varaint"=w30) -> ("error out"=w33:errorcluster)  [unwired: 8 in]
    }
  }
  "error out" <- w27
